vi "AuMT8852B  Initialize.vi"(8 "error in (no error)":errorcluster, 10 "Options":T1={"Reset"=enum."Don't reset", "Identity checking"=enum."Query identity", "Simulation"=enum."Don't simulate", "Range checking"=enum."Don't check attribute ranges", "State caching"=enum."Don't cache attributes", "Status checking"=enum."Query instrument status"}, 11 "GPIB Address (27)":i32=27) -> (0 "error out":errorcluster, 3 "VISA session out":refnum<visa-resource-name>)   [LabVIEW 2017]
doc: "Anritsu MT8852B Bluetooth Tester\n\nOpens a connection to the instrument.\n\nINPUTS\nGPIB address - address on which the instrument is set to receive GPIB commands. For serial connections, use AuMT8850 Initialize.vi.\nOptions - set the behavior of the driver:\nReset: whether or not the driver will reset the instrument to a known state during initialization.\nQuery identity: whether or not the driver will verify that the instrument is an MT8852B before proceeding.\nSimulate: in Simulate mode, the driver will not send any I/O to the instrument.\nCheck attribute ranges: if this setting is turned on, the driver will not send any out-of-range values to the instrument.\nCache attributes: if this setting is turned on, the driver will avoid sending the same command twice.\nQuery instrument status: whether or not the driver will check the instrument for errors after every operation."
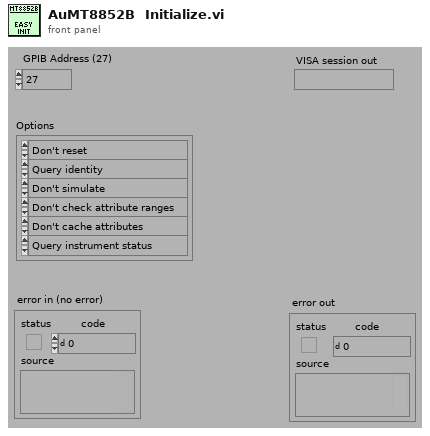
[diagram p1: front panel]
types:
  T1 = cluster{"Reset":enum16{"Don't reset", "Reset"}, "Identity checking":enum16{"Don't query identity", "Query identity"}, "Simulation":enum16{"Don't simulate", "Simulate"}, "Range checking":enum16{"Don't check attribute ranges", "Check attribute ranges"}, "State caching":enum16{"Don't cache attributes", "Cache attributes"}, "Status checking":enum16{"Don't query instrument status", "Query instrument status"}}
  T2 = enum16{"Don't check attribute ranges", "Check attribute ranges"}
  T3 = enum16{"Don't cache attributes", "Cache attributes"}
  T4 = enum16{"Don't query instrument status", "Query instrument status"}
  T5 = cluster{"Simulation":enum16{"Don't simulate", "Simulate"}, "Range checking":enum16{"Don't check attribute ranges", "Check attribute ranges"}, "State caching":enum16{"Don't cache attributes", "Cache attributes"}, "Status checking":enum16{"Don't query instrument status", "Query instrument status"}}
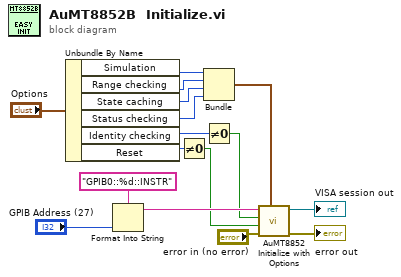
[diagram p0: block diagram]
diagram:
  n1 = Unbundle By Name("Options") -> ("Simulation"=w10:enum16{"Don't simulate", "Simulate"}, "Range checking"=w9:T2, "State caching"=w8:T3, "Status checking"=w7:T4, "Identity checking"=w5:enum16{"Don't query identity", "Query identity"}, "Reset"=w4:enum16{"Don't reset", "Reset"})
  n2 = Format Into String(format string="GPIB0::%d::INSTR" ("Format String"), "GPIB Address (27)") -> (resulting string=w14:string)  [unwired: 2 in, 1 out]
  n3 = Not Equal To 0?(x=w4) -> (x != 0?=w2:bool)
  n4 = Bundle("Simulation"=w10, "Range checking"=w9, "State caching"=w8, "Status checking"=w7) -> (w6:T5)  [unwired: 1 in]
  n5 = Not Equal To 0?(x=w5) -> (x != 0?=w3:bool)
  n6 = call <instrlib>:"AuMT8852 Initialize with Options.vi"("Options"=w6, "error in (no error)"="error in (no error)", "Reset (T)"=w2, "ID Query (T)"=w3, "Resource descriptor (\"GPIB0::27\")"=w14) -> ("error out"=→"error out":errorcluster, "VISA session out"=→"VISA session out":refnum<visa-resource-name>)  [unwired: 5 in]
